vi "Pcre2JitFreeUnusedMemory8.vi"(8 "error in":errorcluster, 11 "pContext":u64 format="%.0x") -> (0 "error out":errorcluster, 3 "pContext":u64 format="%.0x")   [LabVIEW 2021, in "libpcre2-8.lvlib"]
uses:
  libpcre2-8.lvlib
  libpcre2-8-x32.dll
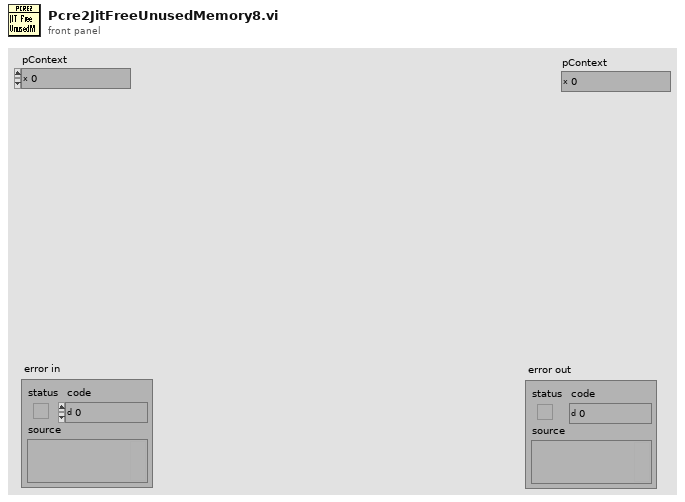
[diagram p1: front panel]
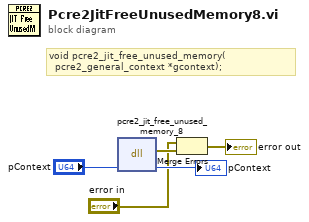
[diagram p0: block diagram]
diagram:
  # "void pcre2_jit_free_unused_memory(\n  pcre2_general_context *gcontext);"
  n1 = dll-call lib="libpcre2-8-x*.dll" fn="pcre2_jit_free_unused_memory_8"("context"="pContext") -> (error out=w3:errorcluster, "context"=→"pContext":u64)  [unwired: 4 in, 1 out]
  n2 = Merge Errors("error in", w3) -> (→"error out":errorcluster)
